vi "One_Tote_Auto.vi"(11 "3_Tote_Enable":bool=TRUE) -> ()   [LabVIEW 2014]
uses:
  General_VI/Global Var.vi
  <vilib>/Rock Robotics/Network Tables/SD Read Number.vi
panel:
  in  "Open_Infeed_time":i32=800
  in  "Extend_Flipper_Time":i32=500
  in  "Time _To_Drive_1_Tote":i32=8000
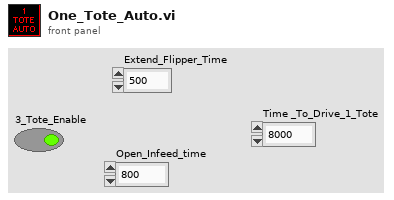
[diagram p1: front panel]
types:
  T1 = cluster{"Open_Infeed_time":i32, "Extend_Flipper_Time":i32, "Time _To_Drive_1_Tote":i32}
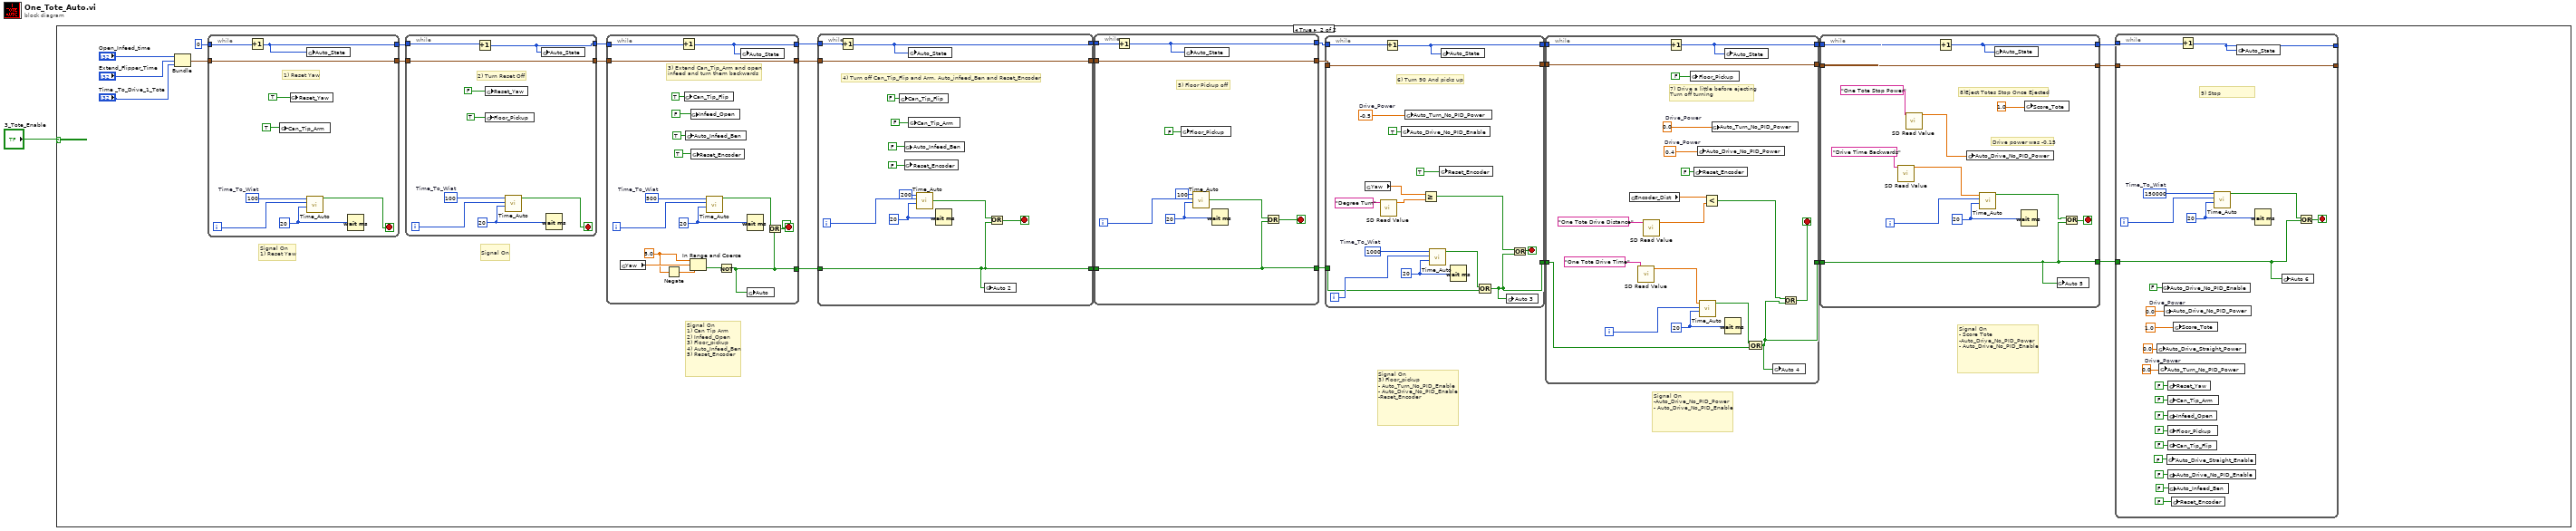
[diagram p0: block diagram]
diagram:
  n1 = case shown="True" "3_Tote_Enable" {
    frame False {
    }
    frame True {
      # "Signal On\n- Score Tote\n-Auto_Drive_No_PID_Power\n- Auto_Drive_No_PID_Enable"
      # "Signal On\n-Auto_Drive_No_PID_Power\n- Auto_Drive_No_PID_Enable"
      # "Signal On\n3) Floor_pickup\n- Auto_Turn_No_PID_Enable\n- Auto_Drive_No_PID_Enable\n-Reset_Encoder"
      # "Signal On\n1) Can Tip Arm\n2) Infeed_Open\n3) Floor_pickup\n4) Auto_Infeed_Ben\n5) Reset_Encoder"
      # "Signal On"
      # "Signal On\n1) Reset Yaw"
      n2 = Bundle("Open_Infeed_time"="Open_Infeed_time", "Extend_Flipper_Time"="Extend_Flipper_Time", "Time _To_Drive_1_Tote"="Time _To_Drive_1_Tote") -> (w19:T1)  [unwired: 1 in]
      n3 = while {
        tunnel: 0 -> [w152]
        tunnel: [w151] -> w27
        tunnel: w19 -> [w153]
        tunnel: [w153] -> w18
        i -> [w156]
        stop <- w158 stop-if-true
        w157 = u32 20 ("milliseconds to wait")
        w155 = 100  # Time_To_Wiat
        # "1) Reset Yaw"
        n4 = Increment(x=w152) -> (x+1=w151:i32)
        n5 = global write "Global Var.vi" "Can_Tip_Arm"(TRUE) -> ()
        n6 = global write "Global Var.vi" "Reset_Yaw"(TRUE) -> ()
        n7 = global write "Global Var.vi" "Auto_State"(w151) -> ()
        n8 = call "Time_Auto.vi"("Sample_Time"=w157, "Counter"=w156, "Time_to_wait"=w155) -> ("Boolean"=w158:bool)  [unwired: 8 in]
        n9 = Wait (ms)(milliseconds to wait=w157) -> ()  [unwired: 1 out]
      }
      n10 = while {
        tunnel: w27 -> [w143]
        tunnel: [w142] -> w26
        tunnel: w18 -> [w144]
        tunnel: [w144] -> w17
        i -> [w147]
        stop <- w149 stop-if-true
        w148 = u32 20 ("milliseconds to wait")
        w146 = 100  # Time_To_Wiat
        # "2) Turn Reset Off"
        n11 = Increment(x=w143) -> (x+1=w142:i32)
        n12 = global write "Global Var.vi" "Floor_Pickup"(TRUE) -> ()
        n13 = global write "Global Var.vi" "Reset_Yaw"(FALSE) -> ()
        n14 = call "Time_Auto.vi"("Sample_Time"=w148, "Counter"=w147, "Time_to_wait"=w146) -> ("Boolean"=w149:bool)  [unwired: 8 in]
        n15 = global write "Global Var.vi" "Auto_State"(w142) -> ()
        n16 = Wait (ms)(milliseconds to wait=w148) -> ()  [unwired: 1 out]
      }
      n17 = while {
        tunnel: w26 -> [w136]
        tunnel: [w135] -> w5
        tunnel: w17 -> [w137]
        tunnel: [w137] -> w6
        tunnel: [w125] -> w7
        i -> [w139]
        stop <- w127 stop-if-true
        w131 = 5.0 ("upper limit")
        w140 = u32 20 ("milliseconds to wait")
        w138 = 500  # Time_To_Wiat
        # "3) Extend Can_Tip_Arm and open \ninfeed and turn them backwards"
        n18 = global read "Global Var.vi" "Yaw"() -> (w133:dbl)
        n19 = Negate(x=w131) -> (-x=w132:dbl)
        n20 = Increment(x=w136) -> (x+1=w135:i32)
        n21 = global write "Global Var.vi" "Can_Tip_Flip"(TRUE ("Can_Tip_Flip")) -> ()
        n22 = global write "Global Var.vi" "Auto_Infeed_Ben"(TRUE) -> ()
        n23 = In Range and Coerce(upper limit=w131, x=w133, lower limit=w132) -> (In Range?=w130:bool)  [unwired: 1 out]
        n24 = global write "Global Var.vi" "Infeed_Open"(FALSE) -> ()
        n25 = global write "Global Var.vi" "Reset_Encoder"(TRUE) -> ()
        n26 = call "Time_Auto.vi"("Sample_Time"=w140, "Counter"=w139, "Time_to_wait"=w138) -> ("Boolean"=w126:bool)  [unwired: 8 in]
        n27 = Not(x=w130) -> (.not. x?=w125:bool)
        n28 = global write "Global Var.vi" "Auto_State"(w135) -> ()
        n29 = Wait (ms)(milliseconds to wait=w140) -> ()  [unwired: 1 out]
        n30 = global write "Global Var.vi" "Auto"(w125) -> ()
        n31 = Or(x=w126, y=w125) -> (x .or. y?=w127:bool)
      }
      n32 = while {
        tunnel: [w39] -> w4
        tunnel: w5 -> [w38]
        tunnel: w6 -> [w37]
        tunnel: [w37] -> w3
        tunnel: w7 -> [w29]
        tunnel: [w29] -> w2
        i -> [w40]
        stop <- w36 stop-if-true
        w41 = u32 20 ("milliseconds to wait")
        # "4) Turn off Can_Tip_Flip and Arm, Auto_infeed_Ben and Reset_Encoder"
        n33 = Increment(x=w38) -> (x+1=w39:i32)
        n34 = global write "Global Var.vi" "Can_Tip_Flip"(FALSE ("Can_Tip_Flip")) -> ()
        n35 = global write "Global Var.vi" "Auto_Infeed_Ben"(FALSE) -> ()
        n36 = global write "Global Var.vi" "Reset_Encoder"(FALSE) -> ()
        n37 = global write "Global Var.vi" "Auto_State"(w39) -> ()
        n38 = global write "Global Var.vi" "Can_Tip_Arm"(FALSE) -> ()
        n39 = call "Time_Auto.vi"("Sample_Time"=w41, "Counter"=w40, "Time_to_wait"=200) -> ("Boolean"=w35:bool)  [unwired: 8 in]
        n40 = Wait (ms)(milliseconds to wait=w41) -> ()  [unwired: 1 out]
        n41 = global write "Global Var.vi" "Auto 2"(w29) -> ()
        n42 = Or(x=w35, y=w29) -> (x .or. y?=w36:bool)
      }
      n43 = while {
        tunnel: [w49] -> w10
        tunnel: w4 -> [w48]
        tunnel: w3 -> [w47]
        tunnel: [w47] -> w9
        tunnel: w2 -> [w44]
        tunnel: [w44] -> w8
        i -> [w50]
        stop <- w46 stop-if-true
        w51 = u32 20 ("milliseconds to wait")
        # "5) Floor Pickup off"
        n44 = Increment(x=w48) -> (x+1=w49:i32)
        n45 = global write "Global Var.vi" "Floor_Pickup"(FALSE) -> ()
        n46 = global write "Global Var.vi" "Auto_State"(w49) -> ()
        n47 = call "Time_Auto.vi"("Sample_Time"=w51, "Counter"=w50, "Time_to_wait"=100) -> ("Boolean"=w45:bool)  [unwired: 8 in]
        n48 = Wait (ms)(milliseconds to wait=w51) -> ()  [unwired: 1 out]
        n49 = Or(x=w45, y=w44) -> (x .or. y?=w46:bool)
      }
      n50 = while {
        tunnel: w10 -> [w122]
        tunnel: [w121] -> w25
        tunnel: w8 -> [w113]
        tunnel: [w109] -> w16
        tunnel: w9 -> [w118]
        tunnel: [w118] -> w13
        i -> [w114]
        stop <- w111 stop-if-true
        w116 = u32 20 ("milliseconds to wait")
        w115 = 1000  # Time_To_Wiat
        w120 = -0.5  # Drive_Power
        # "6) Turn 90 And picks up"
        n51 = global read "Global Var.vi" "Yaw"() -> (w123:dbl)
        n52 = call-poly <vilib>:"SD Read Value.vi"("Name"="Degree Turn") -> ("Numeric"=w108:dbl)  [unwired: 8 in, 2 out]
        n53 = Increment(x=w122) -> (x+1=w121:i32)
        n54 = global write "Global Var.vi" "Auto_Drive_No_PID_Enable"(TRUE ("Auto_Drive_No_PID_Enable")) -> ()
        n55 = global write "Global Var.vi" "Auto_Turn_No_PID_Power"(w120) -> ()
        n56 = Greater Or Equal?(x=w123, y=w108) -> (x >= y?=w110:bool)
        n57 = call "Time_Auto.vi"("Sample_Time"=w116, "Counter"=w114, "Time_to_wait"=w115) -> ("Boolean"=w112:bool)  [unwired: 8 in]
        n58 = global write "Global Var.vi" "Reset_Encoder"(TRUE ("Reset_Encoder")) -> ()
        n59 = global write "Global Var.vi" "Auto_State"(w121) -> ()
        n60 = Wait (ms)(milliseconds to wait=w116) -> ()  [unwired: 1 out]
        n61 = Compound Arithmetic op=OR(w112, w113) -> (w109:bool)
        n62 = global write "Global Var.vi" "Auto 3"(w109) -> ()
        n63 = Or(x=w110, y=w109) -> (x .or. y?=w111:bool)
      }
      n64 = while {
        tunnel: w25 -> [w103]
        tunnel: [w102] -> w24
        tunnel: w16 -> [w97]
        tunnel: [w92] -> w15
        tunnel: w13 -> [w100]
        tunnel: [w100] -> w12
        i -> [w105]
        stop <- w94 stop-if-true
        w101 = 0.0  # Drive_Power
        w104 = 0.4  # Drive_Power
        w106 = u32 20 ("milliseconds to wait")
        # "7) Drive a little before ejecting\nTurn off turning"
        n65 = global read "Global Var.vi" "Encoder_Dist"() -> (w95:dbl)
        n66 = call-poly <vilib>:"SD Read Value.vi"("Name"="One Tote Drive Time") -> ("Numeric"=w88:dbl)  [unwired: 8 in, 2 out]
        n67 = call-poly <vilib>:"SD Read Value.vi"("Name"="One Tote Drive Distance") -> ("Numeric"=w91:dbl)  [unwired: 8 in, 2 out]
        n68 = Increment(x=w103) -> (x+1=w102:i32)
        n69 = global write "Global Var.vi" "Floor_Pickup"(FALSE) -> ()
        n70 = global write "Global Var.vi" "Reset_Encoder"(FALSE ("Reset_Encoder")) -> ()
        n71 = global write "Global Var.vi" "Auto_Drive_No_PID_Power"(w104) -> ()
        n72 = call "Time_Auto.vi"("Sample_Time"=w106, "Counter"=w105, "Time_to_wait"=w88) -> ("Boolean"=w98:bool)  [unwired: 8 in]
        n73 = Less?(x=w95, y=w91) -> (x < y?=w93:bool)
        n74 = global write "Global Var.vi" "Auto_Turn_No_PID_Power"(w101) -> ()
        n75 = global write "Global Var.vi" "Auto_State"(w102) -> ()
        n76 = Wait (ms)(milliseconds to wait=w106) -> ()  [unwired: 1 out]
        n77 = Compound Arithmetic op=OR(w98, w97) -> (w92:bool)
        n78 = global write "Global Var.vi" "Auto 4"(w92) -> ()
        n79 = Or(x=w93, y=w92) -> (x .or. y?=w94:bool)
      }
      n80 = while {
        tunnel: w24 -> [w84]
        tunnel: [w83] -> w23
        tunnel: w15 -> [w79]
        tunnel: [w79] -> w14
        tunnel: w12 -> [w82]
        tunnel: [w82] -> w11
        i -> [w86]
        stop <- w81 stop-if-true
        w87 = u32 20 ("milliseconds to wait")
        # "Drive power was -0.15"
        # "8)Eject Totes Stop Once Ejected"
        n81 = call-poly <vilib>:"SD Read Value.vi"("Name"="Drive Time Backwards") -> ("Numeric"=w77:dbl)  [unwired: 8 in, 2 out]
        n82 = call-poly <vilib>:"SD Read Value.vi"("Name"="One Tote Stop Power") -> ("Numeric"=w75:dbl)  [unwired: 8 in, 2 out]
        n83 = Increment(x=w84) -> (x+1=w83:i32)
        n84 = global write "Global Var.vi" "Auto_Drive_No_PID_Power"(w75) -> ()
        n85 = call "Time_Auto.vi"("Sample_Time"=w87, "Counter"=w86, "Time_to_wait"=w77) -> ("Boolean"=w80:bool)  [unwired: 8 in]
        n86 = global write "Global Var.vi" "Auto_State"(w83) -> ()
        n87 = Wait (ms)(milliseconds to wait=w87) -> ()  [unwired: 1 out]
        n88 = global write "Global Var.vi" "Score_Tote"(1.0) -> ()
        n89 = global write "Global Var.vi" "Auto 5"(w79) -> ()
        n90 = Or(x=w80, y=w79) -> (x .or. y?=w81:bool)
      }
      n91 = while {
        tunnel: w23 -> [w71]
        tunnel: [w70] -> _
        tunnel: w14 -> [w60]
        tunnel: w11 -> [w63]
        tunnel: [w63] -> _
        i -> [w73]
        stop <- w62 stop-if-true
        w53 = 0.0  # Drive_Power
        w57 = 0.0  # Drive_Power
        w74 = u32 20 ("milliseconds to wait")
        w72 = 150000  # Time_To_Wiat
        # "9) Stop"
        n92 = global write "Global Var.vi" "Auto_Drive_Straight_Power"(0.0 ("Auto_Drive_Straight_Power")) -> ()
        n93 = global write "Global Var.vi" "Auto_Turn_No_PID_Power"(w57) -> ()
        n94 = global write "Global Var.vi" "Auto_Drive_No_PID_Enable"(FALSE ("Auto_Drive_No_PID_Enable")) -> ()
        n95 = global write "Global Var.vi" "Auto_Drive_No_PID_Power"(w53) -> ()
        n96 = global write "Global Var.vi" "Auto_Drive_Straight_Enable"(FALSE ("Auto_Drive_Straight_Enable")) -> ()
        n97 = global write "Global Var.vi" "Reset_Yaw"(FALSE ("Reset_Yaw")) -> ()
        n98 = global write "Global Var.vi" "Can_Tip_Arm"(FALSE ("Can_Tip_Arm")) -> ()
        n99 = global write "Global Var.vi" "Infeed_Open"(FALSE ("Infeed_Open")) -> ()
        n100 = global write "Global Var.vi" "Floor_Pickup"(FALSE ("Floor_Pickup")) -> ()
        n101 = global write "Global Var.vi" "Can_Tip_Flip"(FALSE ("Can_Tip_Flip")) -> ()
        n102 = global write "Global Var.vi" "Auto_Drive_No_PID_Enable"(FALSE ("Auto_Drive_No_PID_Enable")) -> ()
        n103 = global write "Global Var.vi" "Auto_Infeed_Ben"(FALSE) -> ()
        n104 = global write "Global Var.vi" "Reset_Encoder"(FALSE) -> ()
        n105 = global write "Global Var.vi" "Score_Tote"(1.0) -> ()
        n106 = Increment(x=w71) -> (x+1=w70:i32)
        n107 = call "Time_Auto.vi"("Sample_Time"=w74, "Counter"=w73, "Time_to_wait"=w72) -> ("Boolean"=w61:bool)  [unwired: 8 in]
        n108 = global write "Global Var.vi" "Auto_State"(w70) -> ()
        n109 = Wait (ms)(milliseconds to wait=w74) -> ()  [unwired: 1 out]
        n110 = global write "Global Var.vi" "Auto 6"(w60) -> ()
        n111 = Or(x=w61, y=w60) -> (x .or. y?=w62:bool)
      }
    }
  }
